vi "Begin.vi"(11 "Image Size":T1=enum."160x120") -> (0 "error out":errorcluster)   [LabVIEW 2012]
doc: "Called before other user functions, this VI is expected to open initial I/O refnums, load in file data, and do all program initialization. Notice that the <B>error out</B> terminal is simply used for data flow. Wiring it to other structures or subVIs ensures that this VI runs first."
uses:
  <vilib>/Rock Robotics/WPI/Camera/WPI_CameraImageSize.ctl
  <vilib>/Rock Robotics/WPI/Camera/WPI_CameraWhite Balance Values.ctl
  <vilib>/Rock Robotics/WPI/Camera/WPI_CameraExposure Values.ctl
  <vilib>/Rock Robotics/WPI/Camera/WPI_CameraFrameRate.ctl
  <vilib>/Rock Robotics/WPI/DriverStation/WPI_DriverStationRobotMode2.ctl
  <vilib>/Rock Robotics/WPI/Joystick/WPI_JoystickDeviceEnum.ctl
  <vilib>/Rock Robotics/SystemInterfaces/DIO/FPGA_DIOPWMChannel.ctl
  <vilib>/Rock Robotics/SystemInterfaces/DIO/FPGA_DIOChannel.ctl
  <vilib>/Rock Robotics/WPI/SafetyOutput/WPI_SafetyOutputConfigMenu.ctl
  Robot Global Data.vi
  <vilib>/Rock Robotics/WPI/RobotDrive/WPI_RobotDriveOpen4MotorWithJaguar.vi
  <vilib>/Rock Robotics/WPI/RobotDrive/WPI_RobotDriveOpen2MotorWithJaguar.vi
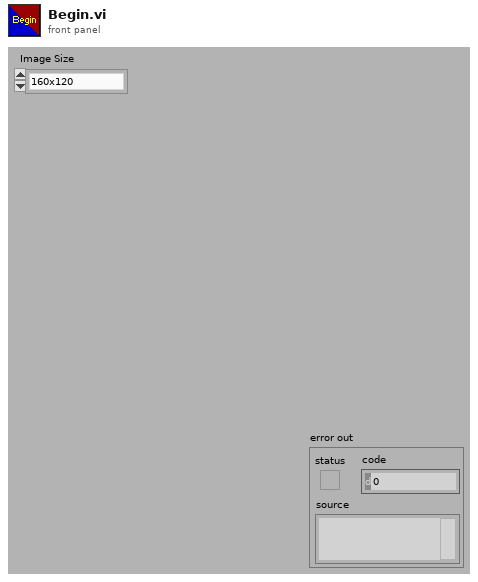
[diagram p1: front panel]
types:
  T1 = typedef "WPI_CameraImageSize.ctl" = enum16{"640x480", "320x240", "160x120"}
  T2 = typedef "FPGA_DIOChannel.ctl" = enum8{"DIO 1", "DIO 2", "DIO 3", "DIO 4", "DIO 5", "DIO 6", "DIO 7", "DIO 8", "DIO 9", "DIO 10", "DIO 11", "DIO 12", "DIO 13", "DIO 14", "Invalid"}
  T3 = typedef "FPGA_DIOPWMChannel.ctl" = enum8{"PWM 1", "PWM 2", "PWM 3", "PWM 4", "PWM 5", "PWM 6", "PWM 7", "PWM 8", "PWM 9", "PWM 10", "Invalid"}
  T4 = typedef "WPI_JoystickDeviceEnum.ctl" = enum16{"USB 1", "USB 2", "USB 3", "USB 4", "Kinect 1", "Kinect 2"}
  T5 = typedef "WPI_DriverStationRobotMode2.ctl" = enum16{"Autonomous Disabled", "Autonomous Enabled", "Teleop Disabled", "Teleop Enabled", "Timeout", "Finish", "Test Disabled", "Test Enabled"}
  T6 = typedef "WPI_CameraFrameRate.ctl" = u32
  T7 = typedef "WPI_CameraExposure Values.ctl" = enum16{"Auto", "Flicker-free 50 Hz", "Flicker-free 60 Hz", "Hold current"}
  T8 = typedef "WPI_CameraWhite Balance Values.ctl" = enum16{"Auto", "Fixed indoor", "Fixed outdoor 1", "Fixed outdoor 2", "Fixed fluorescent 1", "Fixed fluorescent 2", "Hold current"}
  T9 = typedef "WPI_SafetyOutputConfigMenu.ctl" = enum16{"Enable", "Disable"}
  T10 = typedef "WPI_RobotDriveDevRef.ctl" = cluster{"DevStatus":errorcluster, "Motors[]":T11[], "Square Inputs":bool, "Max Output":dbl, "Isochronous":bool}
  T11 = typedef "WPI_MotorControlDeviceRef.ctl" = cluster{"DeviceStatus":errorcluster, "Type":enum16{"PWM", "CAN"}, "PWM":cluster{"Digital Module":T12, "PWM Channel":T3, "DeadBand":T13}, "CAN":cluster{"Device Number":u8, "Control Mode":T14, "Semaphore":T15, "Max Vout":dbl}, "Invert":bool, "TransformRef":T16, "InvTransformRef":T16}
  T12 = typedef "FPGA_TypedefDigitalModule.ctl" = enum16{"Digital Module 1", "Digital Module 2"}
  T13 = typedef "WPI_PWMDeadband.ctl" = cluster{"Name":string, "maxPositivePwm":i32, "minPositivePwm":i32, "centerPwm":i32, "maxNegativePwm":i32, "minNegativePwm":i32, "angularRange":u16}
  T14 = typedef "WPI_CANJaguar_ControlMode.ctl" = enum8{"Percent VBus", "Current", "Speed", "Position", "Voltage"}
  T15 = typedef "Semaphore RefNum" = refnum<k1>
  T16 = typedef "WPI_PWMTransform_ConPane.ctl" = refnum<vi>
  T17 = typedef "WPI_JoystickDevRef.ctl" = cluster{"Device":T4}
  T18 = typedef "WPI_ServoDeviceRef.ctl" = cluster{"DeviceStatus":errorcluster, "Digital Module":T12, "PWM Channel":T3, "DeadBand":T13}
  T19 = typedef "WPI_CameraDevRef.ctl" = cluster{"Camera Address":string, "CameraStatus":errorcluster, "Acquire Image Notifier":refnum<notifier>}
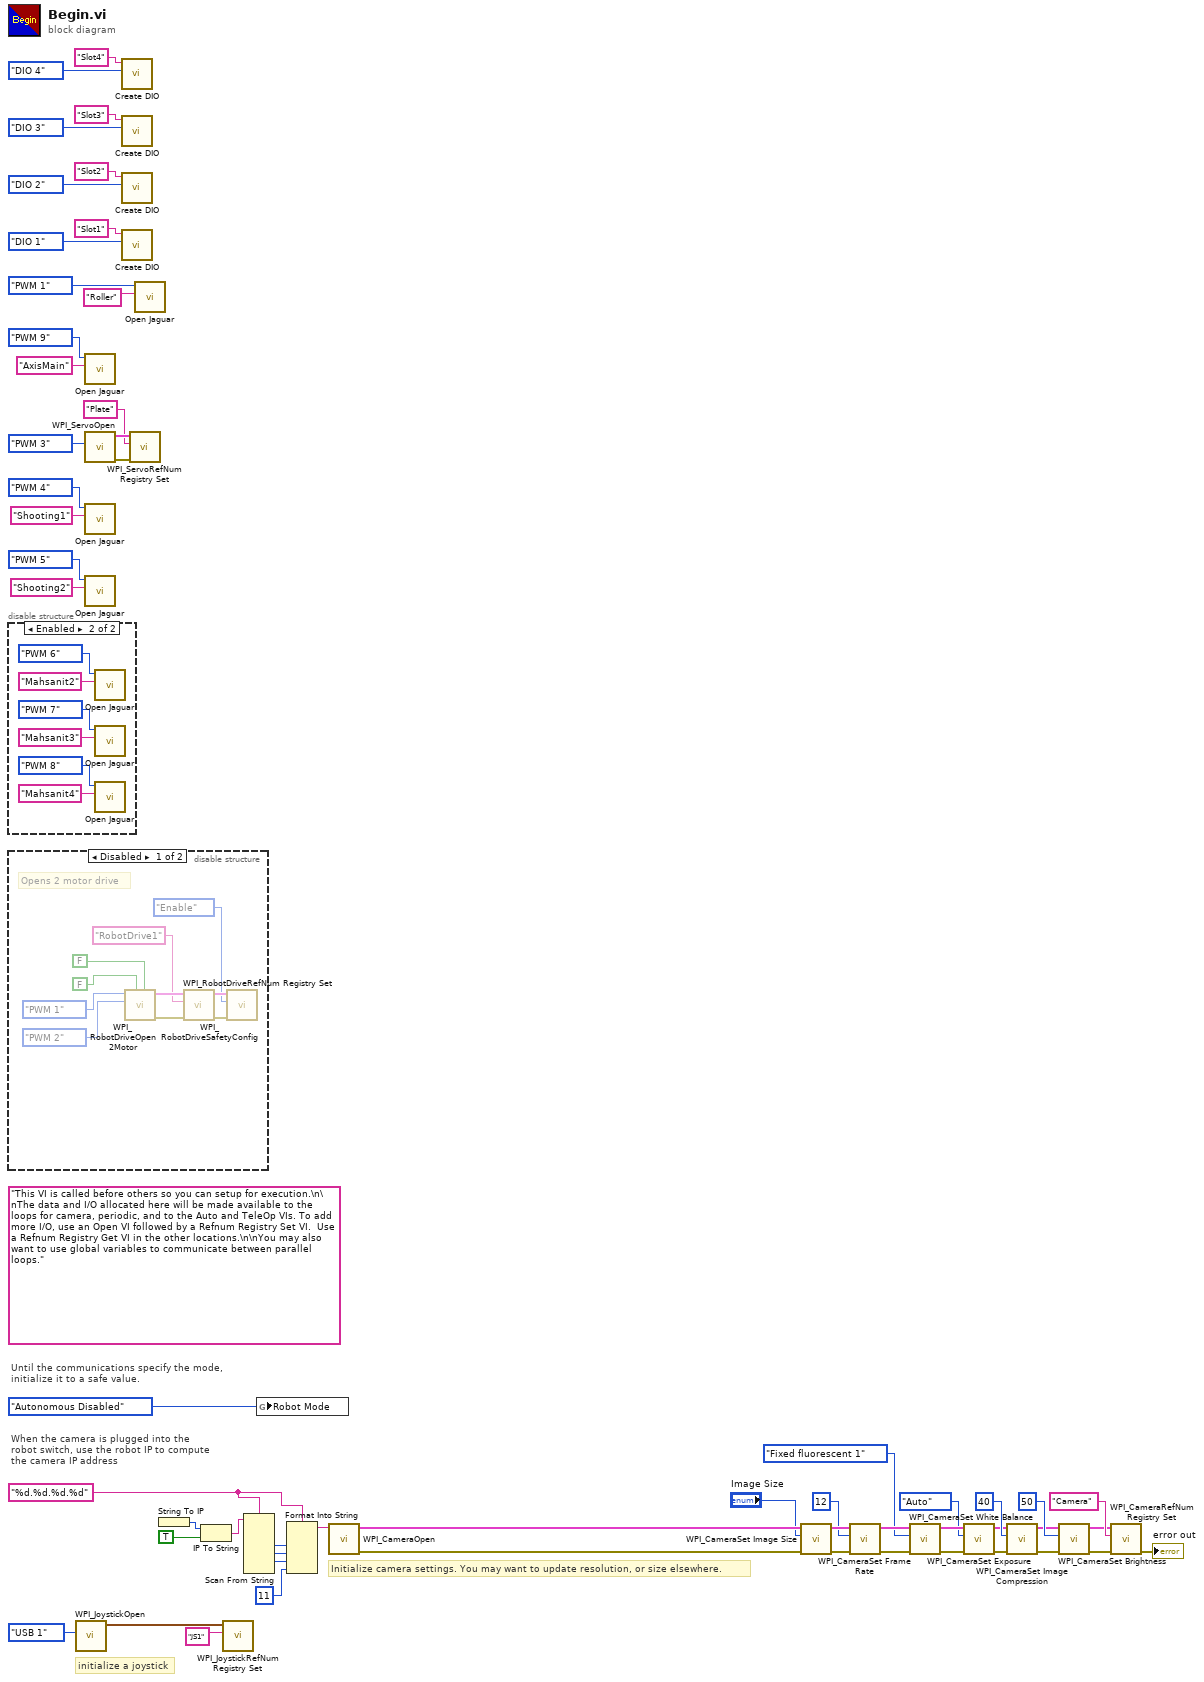
[diagram p0: block diagram]
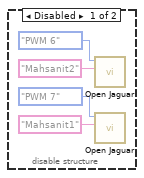
[diagram p2: hidden frame]
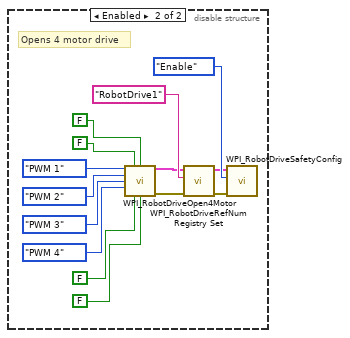
[diagram p3: hidden frame]
diagram:
  w27 = "%d.%d.%d.%d" ("format string")
  (unwired) "This VI is called before others so you can setup for execution.\n\nThe data and I/O allocated here will be made available to the loops for camera, periodic, and to the Auto and TeleOp VIs. To add more I/O, use an Open VI followed by a Refnum Registry Set VI.  Use a Refnum Registry Get VI in the other locations.\n\nYou may also want to use global variables to communicate between parallel loops."
  # "initialize a joystick"
  # "Until the communications specify the mode,\ninitialize it to a safe value."
  # "When the camera is plugged into the\nrobot switch, use the robot IP to compute\nthe camera IP address"
  # "Initialize camera settings. You may want to update resolution, or size elsewhere."
  n1 = disable-structure shown="Enabled" {
    frame Disabled {
      n2 = call "Open Jaguar.vi"("refnum name"="Mahsanit2", "PWM Channel"=FPGA_DIOPWMChannel."PWM 6") -> ()  [unwired: 10 in]
      n3 = call "Open Jaguar.vi"("refnum name"="Mahsanit1", "PWM Channel"=FPGA_DIOPWMChannel."PWM 7") -> ()  [unwired: 10 in]
    }
    frame Enabled {
      n4 = call "Open Jaguar.vi"("refnum name"="Mahsanit2", "PWM Channel"=FPGA_DIOPWMChannel."PWM 6") -> ()  [unwired: 10 in]
      n5 = call "Open Jaguar.vi"("refnum name"="Mahsanit3", "PWM Channel"=FPGA_DIOPWMChannel."PWM 7") -> ()  [unwired: 10 in]
      n6 = call "Open Jaguar.vi"("refnum name"="Mahsanit4", "PWM Channel"=FPGA_DIOPWMChannel."PWM 8") -> ()  [unwired: 10 in]
    }
  }
  n7 = disable-structure shown="Disabled" {
    frame Disabled {
      # "Opens 2 motor drive"
      n8 = call-poly <vilib>:"WPI_RobotDriveOpen2Motor.vi"("Right Motor Inverted"=FALSE, "Left Motor Inverted"=FALSE, "Right Motor"=FPGA_DIOPWMChannel."PWM 2", "Left Motor"=FPGA_DIOPWMChannel."PWM 1") -> ("error out"=w75:errorcluster, "RobotDriveDevRef"=w74:T10)  [unwired: 6 in]
      n9 = call <vilib>:"WPI_RobotDriveRefNum Registry Set.vi"("error in (no error)"=w75, "refnum name"="RobotDrive1", "RobotDriveDevRef"=w74) -> ("error out"=w68:errorcluster, "RobotDriveDevRef"=w67:T10)  [unwired: 7 in]
      n10 = call <vilib>:"WPI_RobotDriveSafetyConfig.vi"("error in (no error)"=w68, "mode"=WPI_SafetyOutputConfigMenu."Enable", "RobotDriveDevRef"=w67) -> ()  [unwired: 7 in, 2 out]
    }
    frame Enabled {
      # "Opens 4 motor drive"
      n11 = call-poly <vilib>:"WPI_RobotDriveOpen4Motor.vi"("Rear Left Motor"=FPGA_DIOPWMChannel."PWM 1", "Rear Left Motor Inverted"=FALSE, "Rear Right Motor Inverted"=FALSE, "Rear Right Motor"=FPGA_DIOPWMChannel."PWM 2", "Front Left Motor"=FPGA_DIOPWMChannel."PWM 3", "Front Right Motor"=FPGA_DIOPWMChannel."PWM 4", "Front Left Motor Inverted"=FALSE, "Front Right Motor Inverted"=FALSE) -> ("RobotDriveDevRef"=w85:T10, "error out"=w84:errorcluster)  [unwired: 6 in]
      n12 = call <vilib>:"WPI_RobotDriveRefNum Registry Set.vi"("error in (no error)"=w84, "refnum name"="RobotDrive1", "RobotDriveDevRef"=w85) -> ("error out"=w87:errorcluster, "RobotDriveDevRef"=w88:T10)  [unwired: 7 in]
      n13 = call <vilib>:"WPI_RobotDriveSafetyConfig.vi"("error in (no error)"=w87, "mode"=WPI_SafetyOutputConfigMenu."Enable", "RobotDriveDevRef"=w88) -> ()  [unwired: 7 in, 2 out]
    }
  }
  n14 = call <vilib>:"WPI_JoystickOpen.vi"("JoystickDevice"=WPI_JoystickDeviceEnum."USB 1") -> ("JoystickDevRef"=w23:T17)  [unwired: 10 in]
  n15 = call "Open Jaguar.vi"("refnum name"="AxisMain", "PWM Channel"=FPGA_DIOPWMChannel."PWM 9") -> ()  [unwired: 10 in]
  n16 = call <vilib>:"WPI_ServoOpen.vi"("PWM Channel"=FPGA_DIOPWMChannel."PWM 3") -> ("error out"=w16:errorcluster, "ServoDeviceRef"=w18:T18)  [unwired: 9 in]
  n17 = call "Open Jaguar.vi"("refnum name"="Shooting1", "PWM Channel"=FPGA_DIOPWMChannel."PWM 4") -> ()  [unwired: 10 in]
  n18 = call "Open Jaguar.vi"("refnum name"="Shooting2", "PWM Channel"=FPGA_DIOPWMChannel."PWM 5") -> ()  [unwired: 10 in]
  n19 = call "Create DIO.vi"("DIO Channel"=FPGA_DIOChannel."DIO 4", "refnum name"="Slot4") -> ()  [unwired: 10 in]
  n20 = call "Create DIO.vi"("DIO Channel"=FPGA_DIOChannel."DIO 3", "refnum name"="Slot3") -> ()  [unwired: 10 in]
  n21 = call "Create DIO.vi"("DIO Channel"=FPGA_DIOChannel."DIO 2", "refnum name"="Slot2") -> ()  [unwired: 10 in]
  n22 = call "Create DIO.vi"("DIO Channel"=FPGA_DIOChannel."DIO 1", "refnum name"="Slot1") -> ()  [unwired: 10 in]
  n23 = call <vilib>:"WPI_ServoRefNum Registry Set.vi"("error in (no error)"=w16, "refnum name"="Plate", "ServoDeviceRef"=w18) -> ()  [unwired: 7 in, 2 out]
  n24 = call "Open Jaguar.vi"("refnum name"="Roller", "PWM Channel"=FPGA_DIOPWMChannel."PWM 1") -> ()  [unwired: 10 in]
  n25 = String To IP() -> (0:w34:u32)  [unwired: 1 in]
  n26 = IP To String(1:TRUE ("dot notation? (F)"), 2:w34) -> (0:w32:string)
  n27 = call <vilib>:"WPI_JoystickRefNum Registry Set.vi"("refnum name"="JS1", "JoystickDevRef"=w23) -> ()  [unwired: 8 in, 2 out]
  n28 = Scan From String(format string=w27, input string=w32) -> (output 1=w31:i32, output 2=w30:i32, output 3=w29:i32)  [unwired: 7 in, 3 out]
  n29 = global write "Robot Global Data.vi" "Robot Mode"(WPI_DriverStationRobotMode2."Autonomous Disabled" ("Robot Mode")) -> ()
  n30 = Format Into String(format string=w27, w31, w30, w29, 11 ("Compression")) -> (resulting string=w25:string)  [unwired: 2 in, 1 out]
  n31 = call <vilib>:"WPI_CameraOpen.vi"("Camera Address"=w25) -> ("error out"=w46:errorcluster, "CameraDevRef"=w47:T19)  [unwired: 1 in, 8 out]
  n32 = call <vilib>:"WPI_CameraSet Image Size.vi"("error in (no error)"=w46, "Image Size"="Image Size", "CameraDevRef"=w47) -> ("error out"=w45:errorcluster, "CameraDevRef Out"=w48:T19)  [unwired: 7 out]
  n33 = call <vilib>:"WPI_CameraSet Frame Rate.vi"("error in (no error)"=w45, "Frame Rate (fps)"=T6 12, "CameraDevRef"=w48) -> ("error out"=w44:errorcluster, "CameraDevRef Out"=w50:T19)  [unwired: 7 out]
  n34 = call <vilib>:"WPI_CameraSet White Balance.vi"("error in (no error)"=w44, "White Balance"=WPI_CameraWhite_Balance_Values."Fixed fluorescent 1", "CameraDevRef"=w50) -> ("error out"=w43:errorcluster, "CameraDevRef Out"=w49:T19)  [unwired: 7 out]
  n35 = call <vilib>:"WPI_CameraSet Exposure.vi"("error in (no error)"=w43, "Exposure"=WPI_CameraExposure_Values."Auto", "CameraDevRef"=w49) -> ("error out"=w42:errorcluster, "CameraDevRef Out"=w52:T19)  [unwired: 7 out]
  n36 = call <vilib>:"WPI_CameraSet Image Compression.vi"("error in (no error)"=w42, "Compression"=40, "CameraDevRef"=w52) -> ("error out"=w41:errorcluster, "CameraDevRef Out"=w51:T19)  [unwired: 7 out]
  n37 = call <vilib>:"WPI_CameraSet Brightness.vi"("error in (no error)"=w41, "Brightness"=50, "CameraDevRef"=w51) -> ("error out"=w39:errorcluster, "CameraDevRef Out"=w40:T19)  [unwired: 7 out]
  n38 = call <vilib>:"WPI_CameraRefNum Registry Set.vi"("error in (no error)"=w39, "refnum name"="Camera", "CameraDevRef"=w40) -> ("error out"=→"error out":errorcluster)  [unwired: 8 out]
